vi "Read Enabled.vi"(8 "error in (no error)":errorcluster, 11 "Robot Event in":refnum<class "Robot Event.lvclass">) -> (0 "error out":errorcluster, 2 "Enabled":bool, 3 "Robot Event out":refnum<class "Robot Event.lvclass">)   [LabVIEW 2019, in "Robot Event.lvclass"]
uses:
  Robot Event.lvclass
  Robot Event.lvclass/Robot Event.ctl
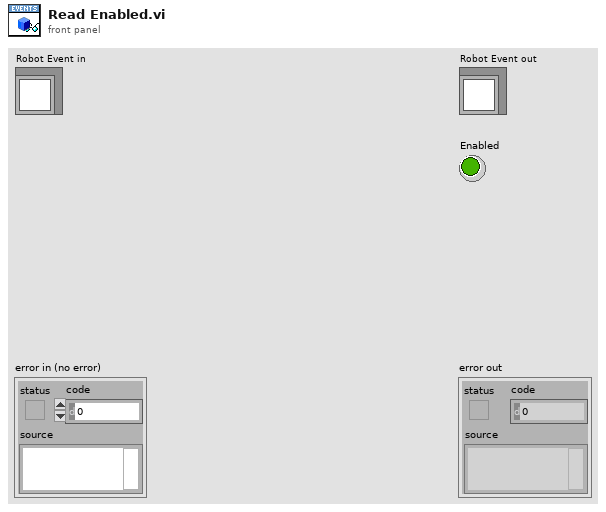
[diagram p1: front panel]
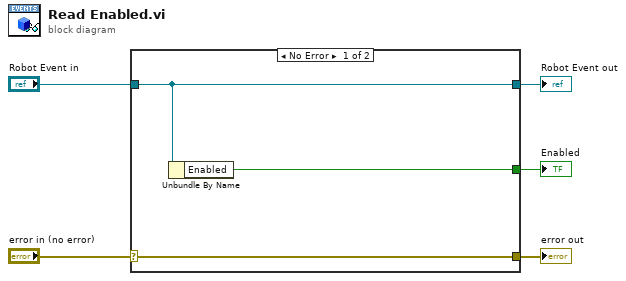
[diagram p0: block diagram]
diagram:
  n1 = case shown="No Error" "error in (no error)" {
    selector: "error in (no error)" -> [w8 w9]
    tunnel: [w8 w9] -> w4
    tunnel: [w7 w10] -> w2
    tunnel: "Robot Event in" -> [w7 w10]
    tunnel: [w6 _] -> w1
    frame No Error {
      n2 = Unbundle By Name(w7) -> ("Enabled"=w6:bool)
    }
    frame Error {
    }
  }
  "error out" <- w4
  "Robot Event out" <- w2
  "Enabled" <- w1
